vi "Initialize.vi"(7 "Parcel Weight [kg]":dbl, 8 "error in (no error)":errorcluster, 9 "Recipient Data":T1, 10 "Sender Data":T1, 11 "Delivery in":refnum<class "Delivery.lvclass">) -> (0 "error out":errorcluster, 3 "Delivery out":refnum<class "Delivery.lvclass">)   [LabVIEW 2019, in "Delivery.lvclass"]
uses:
  Delivery.lvclass
  Controls/#cluster_PersonalData.ctl
  Delivery.lvclass/Delivery.ctl
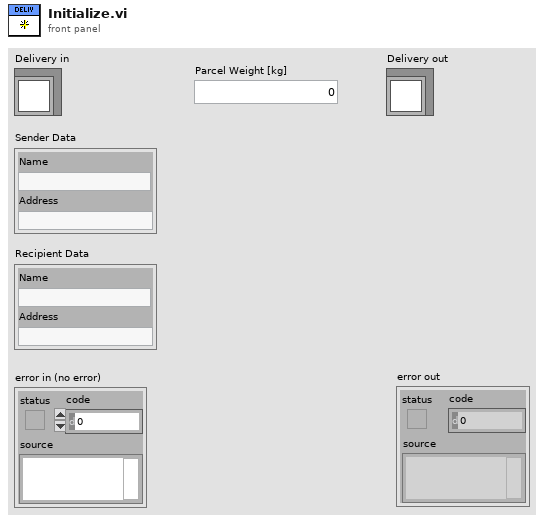
[diagram p1: front panel]
types:
  T1 = typedef "#cluster_PersonalData.ctl" = cluster{"Name":string, "Address":string}
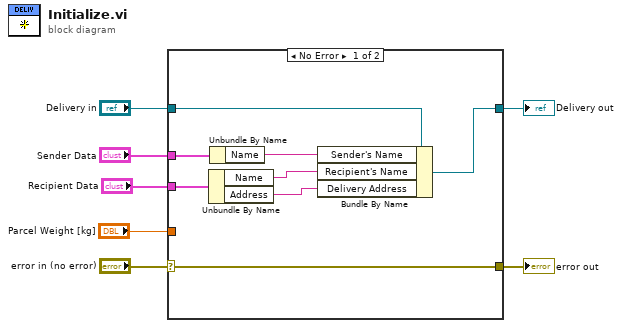
[diagram p0: block diagram]
diagram:
  n1 = case shown="No Error" "error in (no error)" {
    selector: "error in (no error)" -> [w15 w17]
    tunnel: [w15 w17] -> w6
    tunnel: [w13 w16] -> w4
    tunnel: "Delivery in" -> [w14 w16]
    tunnel: "Sender Data" -> [w12 _]
    tunnel: "Recipient Data" -> [w11 _]
    tunnel: "Parcel Weight [kg]" -> [_ _]
    frame No Error {
      n2 = Unbundle By Name(w11) -> ("Name"=w9:string, "Address"=w8:string)
      n3 = Unbundle By Name(w12) -> ("Name"=w10:string)
      n4 = Bundle By Name(cluster=w14, "Sender's Name"=w10, "Recipient's Name"=w9, "Delivery Address"=w8) -> (w13:refnum<class "Delivery.lvclass">)
    }
    frame Error {
    }
  }
  "error out" <- w6
  "Delivery out" <- w4
